vi "Get JSON Type From LV Type.vi"(11 "Labview Datatype":T1) -> (0 "error out":errorcluster, 3 "JSON Schema Type":string)   [LabVIEW 2020, in "JSON Schema Generator.lvlib"]
uses:
  JSON Schema Generator.lvlib
  <vilib>/Utility/Data Type/Type Definitions/Data Type.ctl
  <userlib>/_OpenG.lib/error/error.llb/openg_error.lvlib
  <vilib>/Utility/Data Type/NI_Data Type.lvlib
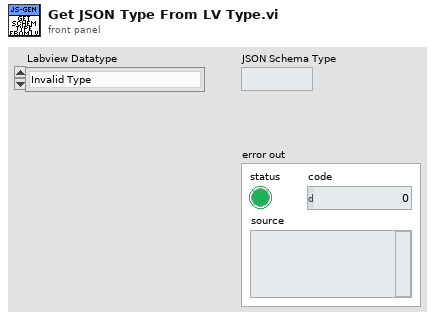
[diagram p1: front panel]
types:
  T1 = typedef "NI_Data Type.lvlib/Data Type.ctl" = enum8{"Invalid Type", "Void", "I8", "I16", "I32", "I64", "U8", "U16", "U32", "U64", "Single Float", "Double Float", "Extended Float", "Single Complex", "Double Complex", "Extended Complex", "Enum U8", "Enum U16", "Enum U32", "Enum U64", "Single Float With Unit", "Double Float With Unit", "Extended Float With Unit", "Single Complex with Unit", "Double Complex with Unit", "Extended Complex with Unit", "Boolean", "String", "Path", "Picture", "Tag", "Array", "Cluster", "Variant", "LV Variant", "Waveform", "Timestamp", "Digital Waveform", "Digital Data", "ExpressData", "Refnum", "External Data", "VI", "Poly VI", "LabVIEW Class Instance", "Fixed Point", "Set Collection", "Map Collection"}
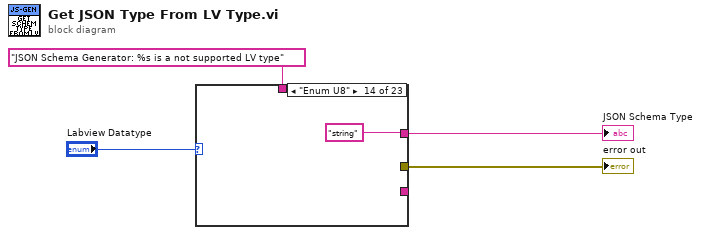
[diagram p0: block diagram]
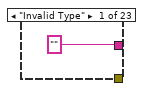
[diagram p2: hidden frame]
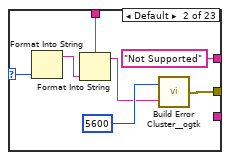
[diagram p3: hidden frame]
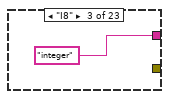
[diagram p4: hidden frame]
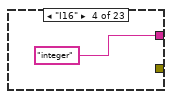
[diagram p5: hidden frame]
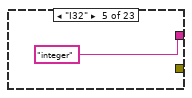
[diagram p6: hidden frame]
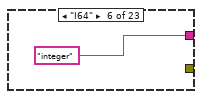
[diagram p7: hidden frame]
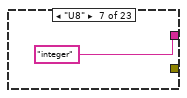
[diagram p8: hidden frame]
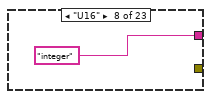
[diagram p9: hidden frame]
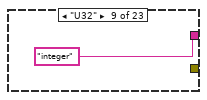
[diagram p10: hidden frame]
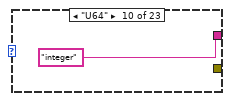
[diagram p11: hidden frame]
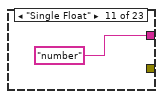
[diagram p12: hidden frame]
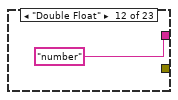
[diagram p13: hidden frame]
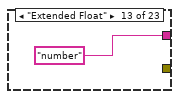
[diagram p14: hidden frame]
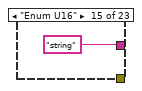
[diagram p15: hidden frame]
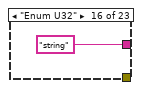
[diagram p16: hidden frame]
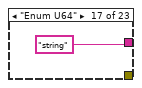
[diagram p17: hidden frame]
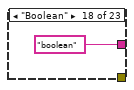
[diagram p18: hidden frame]
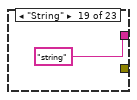
[diagram p19: hidden frame]
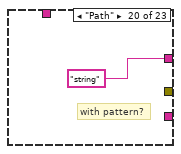
[diagram p20: hidden frame]
diagram:
  n1 = case shown="\"Enum U8\"" "Labview Datatype" {
    selector: "Labview Datatype" -> [_ w11 _ _ _ _ _ _ _ _ _ _ _ _ _ _ _ _ _ _ _ _ _]
    tunnel: ["" ("type") "Not Supported" ("type") "integer" "integer" "integer" "integer" "integer" "integer" "integer" "integer" "number" "number" "number" "string" ("type") "string" ("type") "string" ("type") "string" ("type") "boolean" "string" "string" "array" "object" w34] -> w2
    tunnel: [_ w10 _ _ _ _ _ _ _ _ _ _ _ _ _ _ _ _ _ _ _ _ _] -> w3
    tunnel: "JSON Schema Generator: %s is a not supported LV type" ("String to Prepend to source (\"\")") -> [_ w9 _ _ _ _ _ _ _ _ _ _ _ _ _ _ _ _ _ _ _ _ _]
    tunnel: [_ _ _ _ _ _ _ _ _ _ _ _ _ _ _ _ _ _ _ _ _ _ w33] -> _
    frame "Invalid Type" {
    }
    frame Default {
      n2 = Format Into String(w11) -> (resulting string=w8:string)  [unwired: 3 in, 1 out]
      n3 = Format Into String(format string=w9, w8) -> (resulting string=w7:string)  [unwired: 2 in, 1 out]
      n4 = call <userlib>:"Build Error Cluster__ogtk.vi"("String to Prepend to source (\"\")"=w7, "code"=5600) -> ("error out"=w10:errorcluster)
    }
    frame "I8" {
    }
    frame "I16" {
    }
    frame "I32" {
    }
    frame "I64" {
    }
    frame "U8" {
    }
    frame "U16" {
    }
    frame "U32" {
    }
    frame "U64" {
    }
    frame "Single Float" {
    }
    frame "Double Float" {
    }
    frame "Extended Float" {
    }
    frame "Enum U8" {
    }
    frame "Enum U16" {
    }
    frame "Enum U32" {
    }
    frame "Enum U64" {
    }
    frame "Boolean" {
    }
    frame "String" {
    }
    frame "Path" {
      # "with pattern?"
    }
    frame "Array" {
    }
    frame "Cluster" {
    }
    frame "Timestamp" {
      w33 = "string"  # pattern
      w34 = "string"  # type
    }
  }
  "JSON Schema Type" <- w2
  "error out" <- w3
